vi "Event Actor Wrapper.vi"(4 "Queue Nested":map{string, refnum<data-value>}(c390), 6 "Queue Self":map{string, refnum<data-value>}(c390), 8 "Queue Caller":map{string, refnum<data-value>}(c390), 9 "Queue of Event Self":refnum<queue>, 10 "Event Self Alias":string, 11 "Event jettl":refnum<class "Event jettl.lvclass">) -> ()   [LabVIEW 2021, in "jettl.lvlib" / "Base Event jettl.lvlib"]
uses:
  Base Event jettl.lvlib
  Event jettl/Event jettl.lvclass
  Msg Strategy/Msg Strategy/Msg Strategy.lvclass
  Base Event jettl/Base Event jettl.lvclass
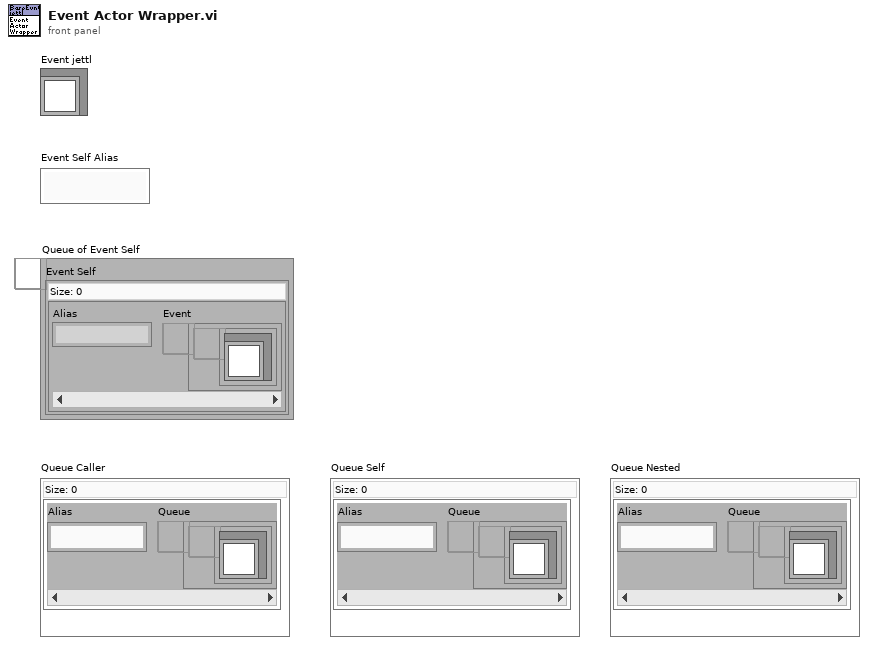
[diagram p1: front panel]
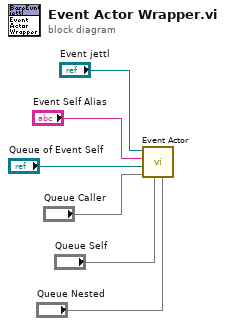
[diagram p0: block diagram]
diagram:
  n1 = call "Event Actor.vi"("Queue Nested"="Queue Nested", "Queue Self"="Queue Self", "Queue Caller"="Queue Caller", "Queue of Event Self"="Queue of Event Self", "Event Self Alias"="Event Self Alias", "Event jettl"="Event jettl") -> ()  [unwired: 6 in]
